vi "AP_2_pulse_control.vi"() -> ()   [LabVIEW 2023]
uses:
  <instrlib>/Quantum Composers 9000 Series/Public/Configure/Configure Chan Mode (Normal).vi
  <instrlib>/Quantum Composers 9000 Series/Quantum Composers 9000 Series.lvlib
panel:
  in  "Gas Pulse Enabled?":bool=TRUE
  in  "Mass Gate Enabled?":bool=TRUE
  in  "Initialization Type":string(combo)="Load from variables "
  in  "Load Conditions":bool
  in  "Save Conditions":bool
  in  "Detachment Laser On?":bool=TRUE
  in  "Detachment Laser Delay / us":dbl=500.0
  in  "Laser In Use":string(combo)="QuantaRay 170-30"
  in  "stop":bool
  in  "Mass Gate Width / us":dbl=0.5 format="%#_3f"
  in  "Mass Gate Delay / us":dbl=85.0
  in  "Repeller Delay / us":dbl=80.0
  # "AP2 Delay Controls"
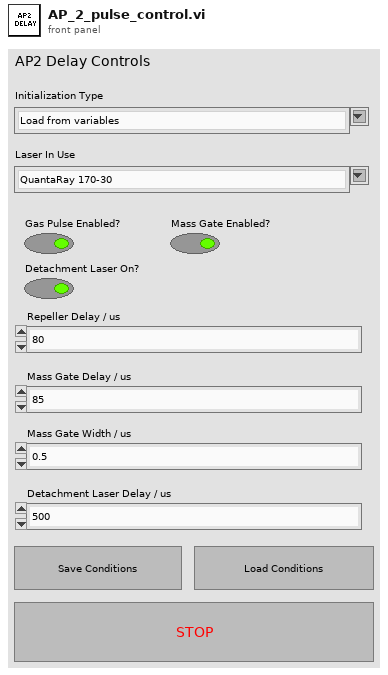
[diagram p1: front panel]
types:
  T1 = cluster{"Mass Gate Delay / us":refnum<vi>, "Mass Gate Width / us":refnum<vi>, "Repeller Delay / us":refnum<vi>, "Mass Gate Enabled?":refnum<vi>, "Gas Pulse Enabled?":refnum<vi>, "Detachment Laser On?":refnum<vi>, "Detachment Laser Delay / us":refnum<vi>}
  T2 = cluster{"Mass Gate Delay / us":dbl, "Mass Gate Width / us":dbl, "Repeller Delay / us":dbl, "Detachment Laser Delay / us":dbl, "Mass Gate Enabled?":bool, "Gas Pulse Enabled?":bool, "Detachment Laser On?":bool}
  T3 = enum16{"Disabled", "Pulse Inhibit", "Output Inhibit"}
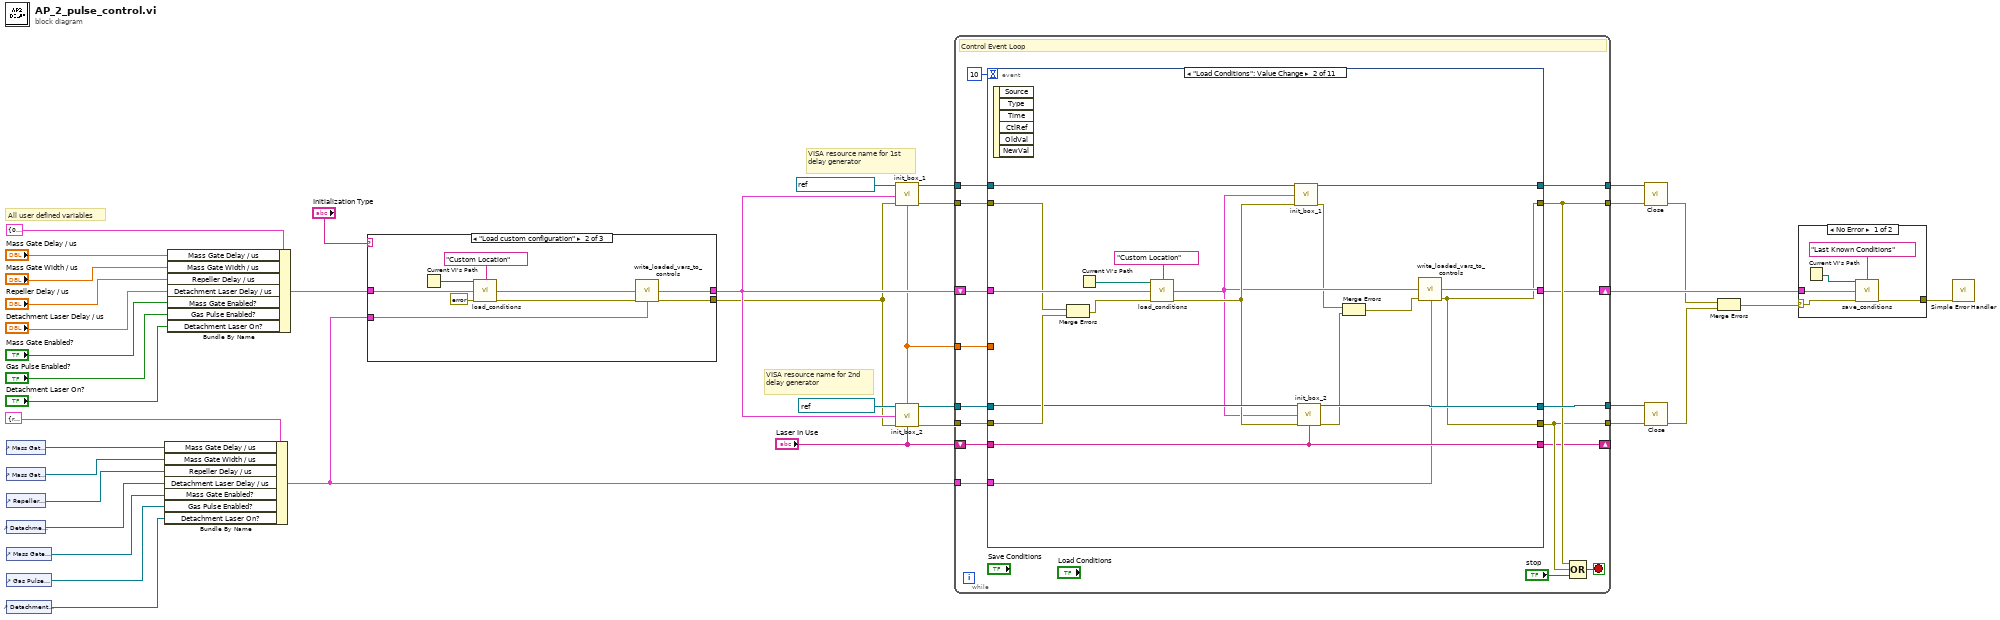
[diagram p0: block diagram]
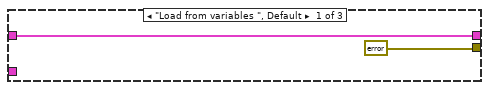
[diagram p2: hidden frame]
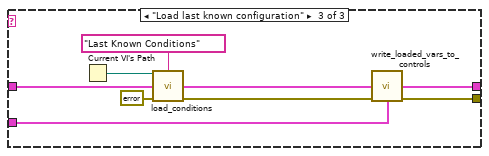
[diagram p3: hidden frame]
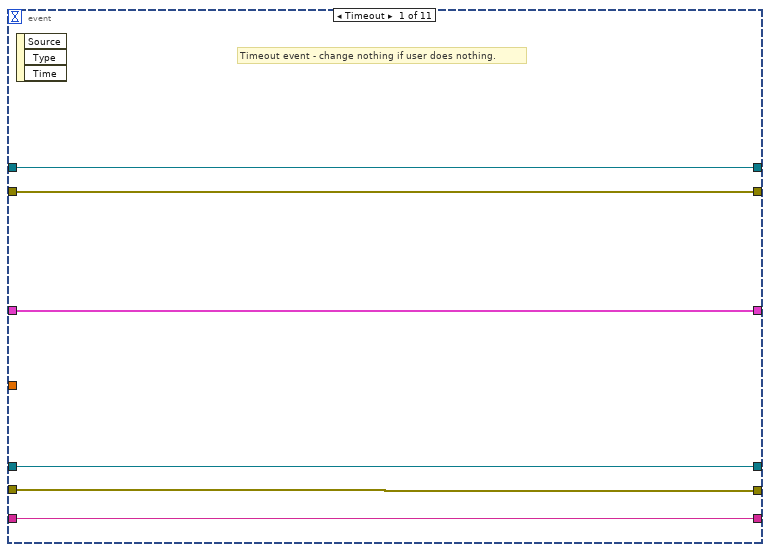
[diagram p5: hidden frame]
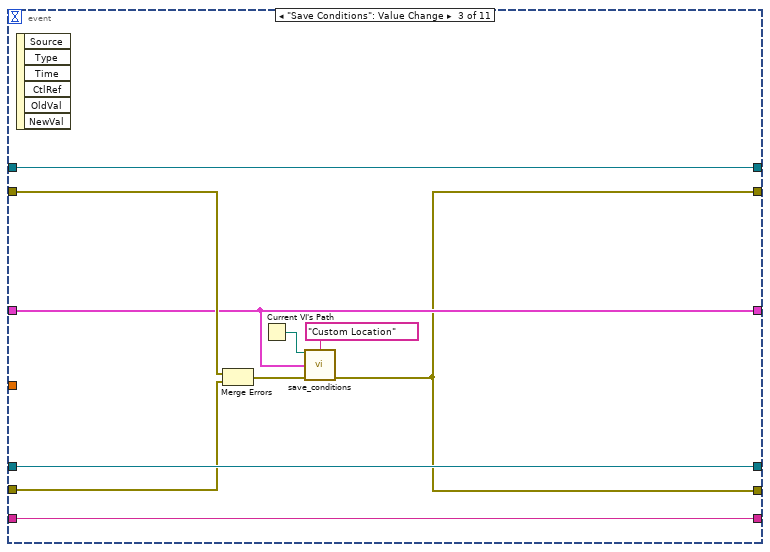
[diagram p6: hidden frame]
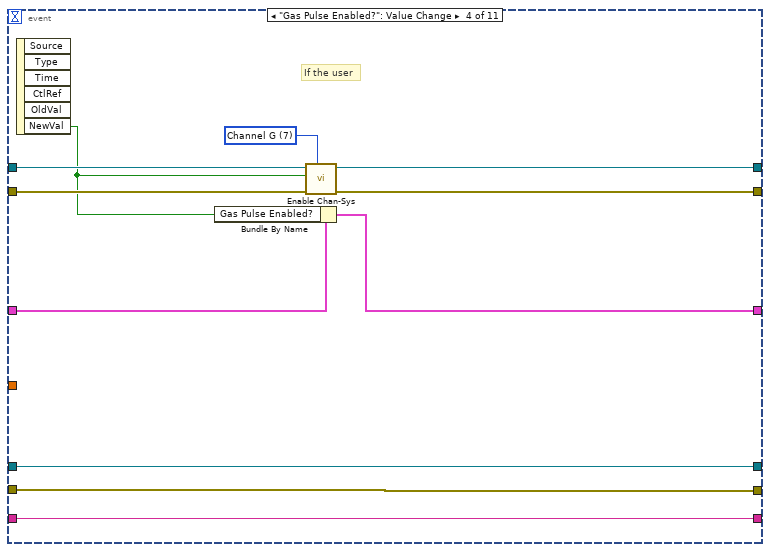
[diagram p7: hidden frame]
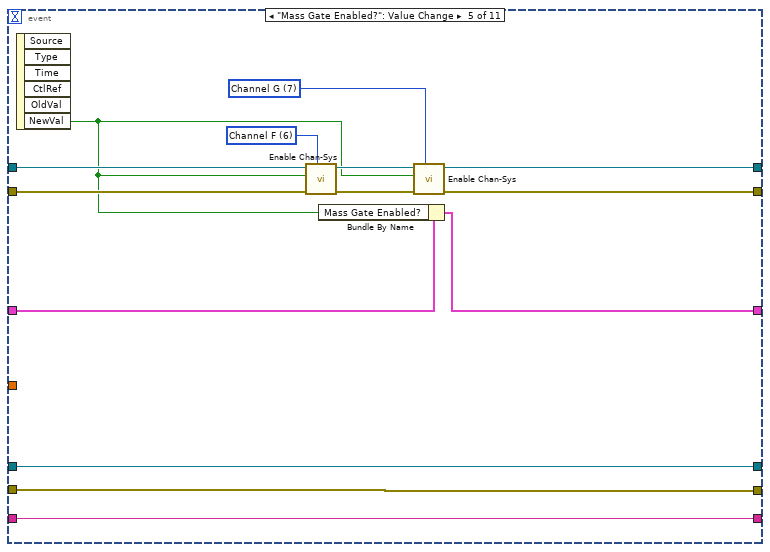
[diagram p8: hidden frame]
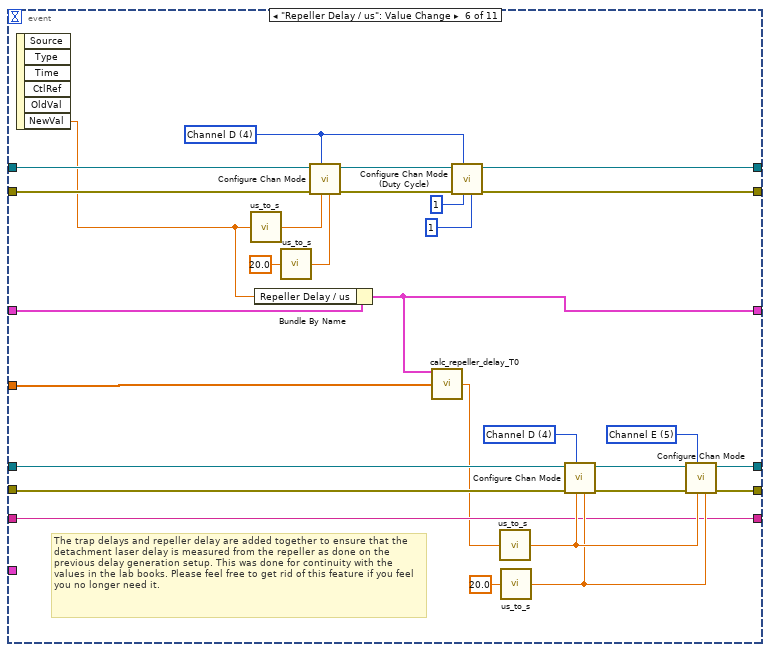
[diagram p9: hidden frame]
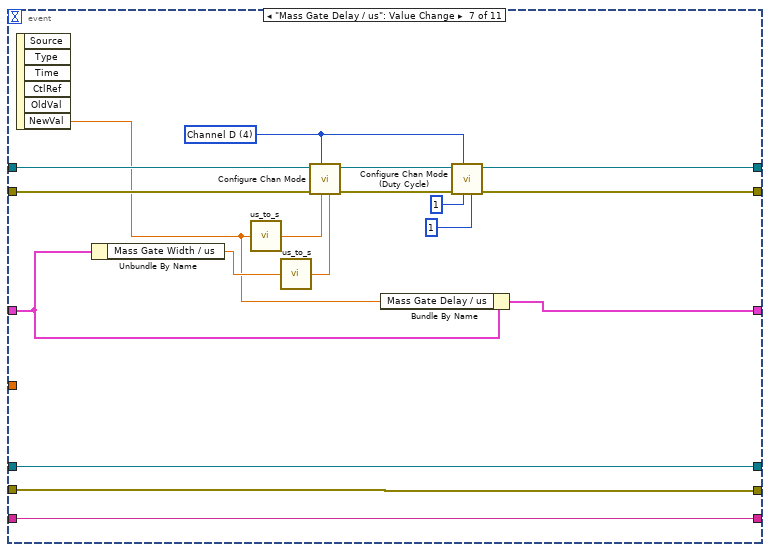
[diagram p10: hidden frame]
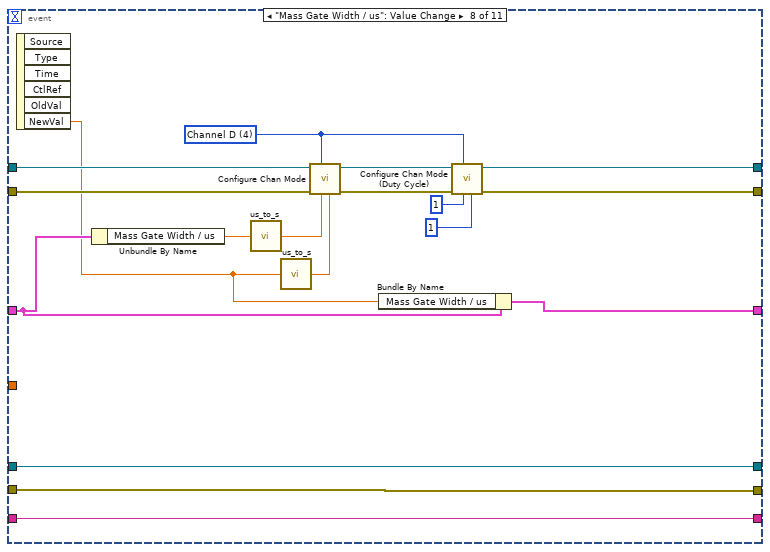
[diagram p11: hidden frame]
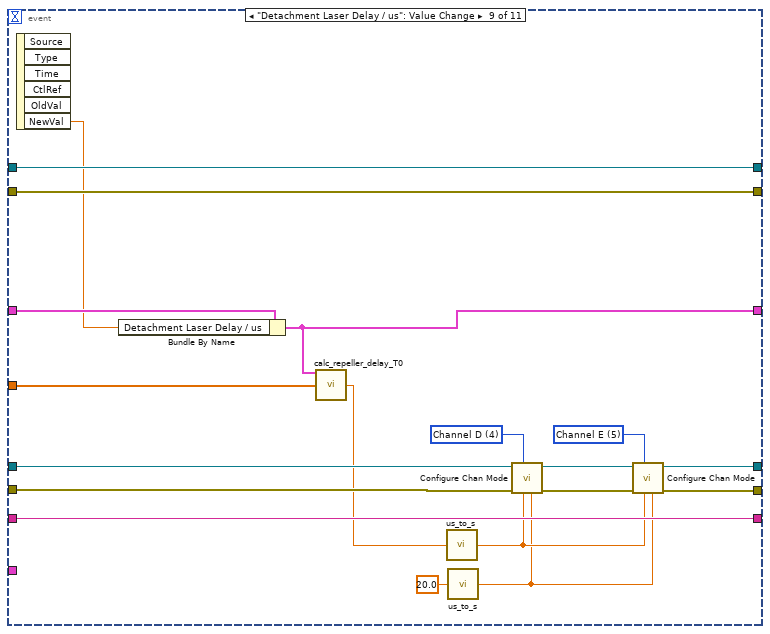
[diagram p12: hidden frame]
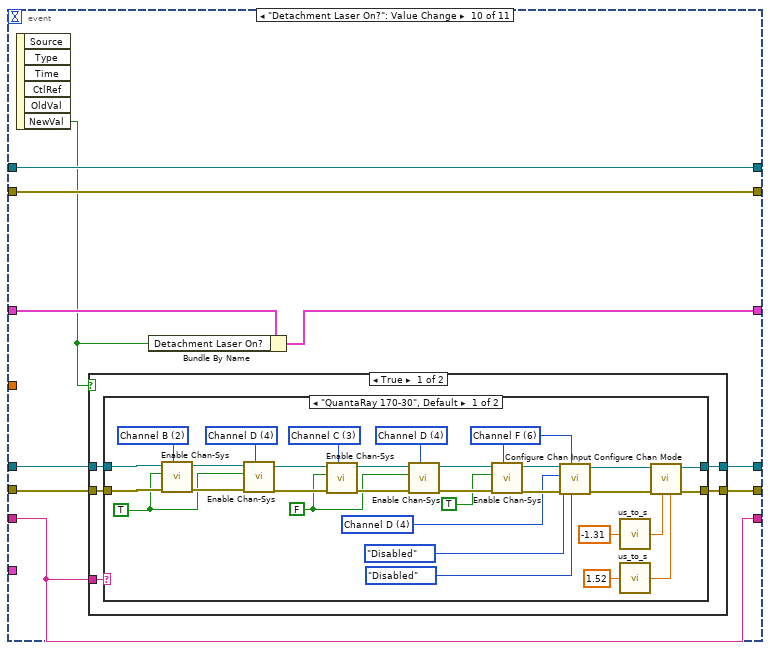
[diagram p13: hidden frame]
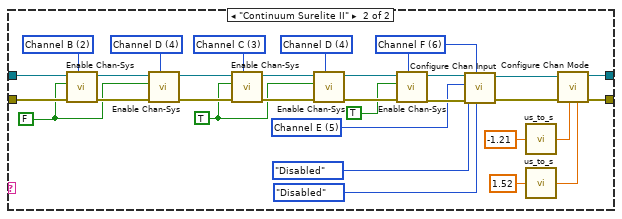
[diagram p14: hidden frame]
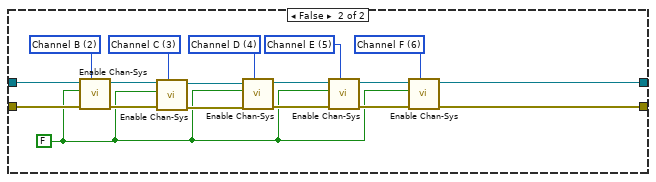
[diagram p15: hidden frame]
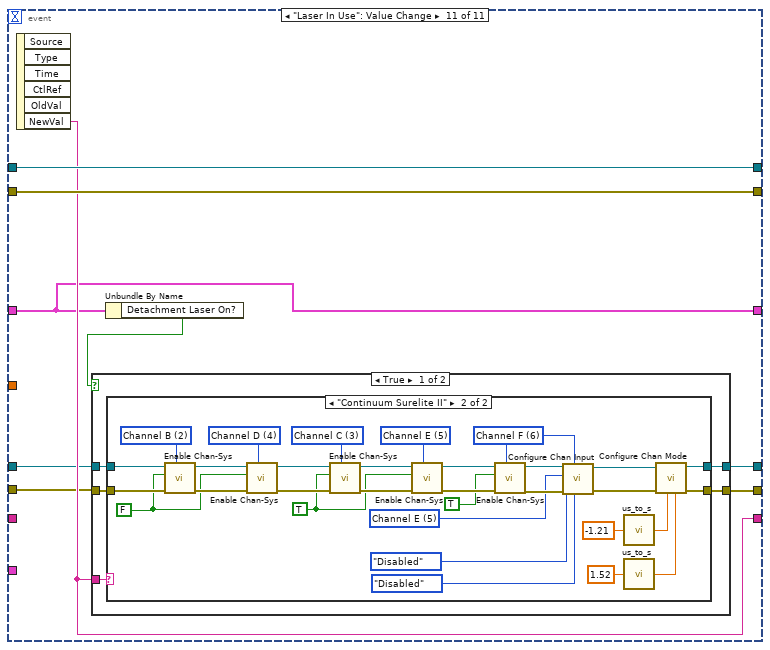
[diagram p16: hidden frame]
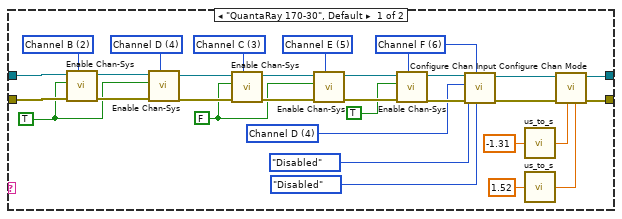
[diagram p17: hidden frame]
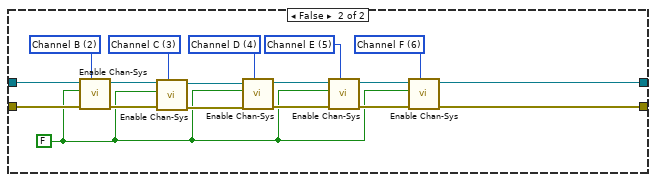
[diagram p18: hidden frame]
diagram:
  # "VISA resource name for 2nd delay generator"
  # "VISA resource name for 1st delay generator"
  # "All user defined variables"
  n1 = control-ref of="Mass Gate Delay / us"() -> (w12:refnum<vi>)
  n2 = control-ref of="Mass Gate Width / us"() -> (w11:refnum<vi>)
  n3 = control-ref of="Repeller Delay / us"() -> (w10:refnum<vi>)
  n4 = control-ref of="Detachment Laser Delay / us"() -> (w9:refnum<vi>)
  n5 = control-ref of="Mass Gate Enabled?"() -> (w2:refnum<vi>)
  n6 = control-ref of="Gas Pulse Enabled?"() -> (w1:refnum<vi>)
  n7 = control-ref of="Detachment Laser On?"() -> (w8:refnum<vi>)
  n8 = Bundle By Name(cluster=T1 {"Mass Gate Delay / us"=refnum, "Mass Gate Width / us"=refnum, "Repeller Delay / us"=refnum, "Mass Gate Enabled?"=refnum, "Gas Pulse Enabled?"=refnum, "Detachment Laser On?"=refnum, "Detachment Laser Delay / us"=refnum}, "Mass Gate Delay / us"=w12, "Mass Gate Width / us"=w11, "Repeller Delay / us"=w10, "Detachment Laser Delay / us"=w9, "Mass Gate Enabled?"=w2, "Gas Pulse Enabled?"=w1, "Detachment Laser On?"=w8) -> (w6:T1)
  n9 = Bundle By Name(cluster=T2 {"Mass Gate Delay / us"=0.0, "Mass Gate Width / us"=0.0, "Repeller Delay / us"=0.0, "Detachment Laser Delay / us"=500.0, "Mass Gate Enabled?"=TRUE, "Gas Pulse Enabled?"=TRUE, "Detachment Laser On?"=FALSE}, "Mass Gate Delay / us"="Mass Gate Delay / us", "Mass Gate Width / us"="Mass Gate Width / us", "Repeller Delay / us"="Repeller Delay / us", "Detachment Laser Delay / us"="Detachment Laser Delay / us", "Mass Gate Enabled?"="Mass Gate Enabled?", "Gas Pulse Enabled?"="Gas Pulse Enabled?", "Detachment Laser On?"="Detachment Laser On?") -> (w16:T2)
  n10 = case shown="\"Load custom configuration\"" "Initialization Type" {
    tunnel: w16 -> [w40 w49 w58]
    tunnel: [w40 w45 w54] -> w15
    tunnel: w6 -> [_ w46 w55]
    tunnel: [errorcluster {"status"=FALSE, "code"=0, "source"=""} ("error in") w43 w52] -> w7
    frame "Load from variables ", Default {
    }
    frame "Load custom configuration" {
      n11 = Current VI's Path() -> (path=w42:path)
      n12 = call "load_conditions.vi"("VI's Path"=w42, "Load Type"="Custom Location", "Config In"=w49, "error in"=errorcluster {"status"=FALSE, "code"=0, "source"=""}) -> ("Config Out"=w48:T2, "error out"=w47:errorcluster)  [unwired: 10 in]
      n13 = call "write_loaded_vars_to_controls.vi"("Variable Values"=w48, "error in (no error)"=w47, "Variable References"=w46) -> ("Variable Values Out"=w45:T2, "error out"=w43:errorcluster)  [unwired: 11 in]
    }
    frame "Load last known configuration" {
      n14 = Current VI's Path() -> (path=w51:path)
      n15 = call "load_conditions.vi"("VI's Path"=w51, "Load Type"="Last Known Conditions", "Config In"=w58, "error in"=errorcluster {"status"=FALSE, "code"=0, "source"=""}) -> ("Config Out"=w57:T2, "error out"=w56:errorcluster)  [unwired: 10 in]
      n16 = call "write_loaded_vars_to_controls.vi"("Variable Values"=w57, "error in (no error)"=w56, "Variable References"=w55) -> ("Variable Values Out"=w54:T2, "error out"=w52:errorcluster)  [unwired: 11 in]
    }
  }
  n17 = call "init_box_1.vi"("Box I VISA Name"=refnum<visa-resource-name> "QC_9530_DG1", "Controls Cluster"=w15, "error in (no error)"=w7) -> ("Box I VISA Name"=w34:refnum<visa-resource-name>, "Trap Delay Array"=w5:dbl[], "error out"=w33:errorcluster)  [unwired: 10 in]
  n18 = call "init_box_2.vi"("Box 2 VISA Name"=refnum<visa-resource-name> "QC_9530_DG2" ("Box I VISA Name"), "Trap Delay Array"=w5, "Controls Cluster"=w15, "error in (no error)"=w7, "Laser In Use"="Laser In Use") -> ("Box 2 VISA Name Out"=w25:refnum<visa-resource-name>, "Error out"=w24:errorcluster)  [unwired: 9 in]
  n19 = while {
    tunnel: w34 -> [w75]
    tunnel: w33 -> [w74]
    tunnel: [w73] -> w38
    tunnel: [w68] -> w37
    tunnel: w25 -> [w71]
    tunnel: w24 -> [w70]
    tunnel: [w69] -> w36
    tunnel: [w67] -> w35
    shift-right: [w63] -> w21
    shift-left: w15 -> [w64]
    shift-right: [w61] -> _
    shift-left: "Laser In Use" -> [w62]
    tunnel: w6 -> [w60]
    tunnel: w5 -> [w59]
    stop <- w66 stop-if-true
    # "Control Event Loop"
    n20 = event shown="[1] \"Load Conditions\": Value Change" {
      selector: _ -> [_ _ _ _ _ _ _ _ _ _ _]
      dyn-events: _ -> [_ _ _ _ _ _ _ _ _ _ _]
      timeout: 10 -> [_ _ _ _ _ _ _ _ _ _ _]
      tunnel: w75 -> [w81 w99 w110 w118 w132 w164 w180 w198 w219 w229 w323]
      tunnel: w74 -> [w80 w98 w106 w117 w131 w163 w179 w197 w218 w228 w322]
      tunnel: [w81 w91 w110 w116 w125 w160 w176 w194 w219 w229 w323] -> w73
      tunnel: [w80 w84 w101 w115 w124 w159 w175 w193 w218 w228 w322] -> w68
      tunnel: w71 -> [w79 w94 w109 w121 w135 w144 w182 w200 w217 w224 w318]
      tunnel: w70 -> [w78 w97 w107 w120 w134 w143 w181 w199 w216 w223 w317]
      tunnel: [w79 w95 w109 w121 w135 w142 w182 w200 w207 w222 w321] -> w69
      tunnel: [w78 w84 w101 w120 w134 w141 w181 w199 w206 w221 w320] -> w67
      tunnel: w64 -> [w77 w100 w104 w114 w130 w138 w169 w187 w214 w227 w315]
      tunnel: [w77 w90 w104 w113 w129 w136 w168 w186 w202 w226 w315] -> w63
      tunnel: w62 -> [w76 w92 w108 w119 w133 w140 w165 w183 w215 w220 _]
      tunnel: [w76 w92 w108 w119 w133 w140 w165 w183 w215 w220 w319] -> w61
      tunnel: w60 -> [_ w85 _ _ _ _ _ _ _ _ _]
      tunnel: w59 -> [_ _ _ _ _ w139 _ _ w203 _ _]
      event Timeout {
        # "Timeout event - change nothing if user does nothing."
        n21 = event-data() -> ()  [unwired: 1 in, 3 out]
      }
      event "Load Conditions": Value Change {
        n22 = event-data() -> ()  [unwired: 1 in, 6 out]
        n23 = Merge Errors(w98, w97) -> (w96:errorcluster)
        n24 = Current VI's Path() -> (path=w83:path)
        n25 = call "load_conditions.vi"("VI's Path"=w83, "Load Type"="Custom Location", "Config In"=w100, "error in"=w96) -> ("Config Out"=w89:T2, "error out"=w93:errorcluster)  [unwired: 10 in]
        n26 = call "init_box_1.vi"("Box I VISA Name"=w99, "Controls Cluster"=w89, "error in (no error)"=w93) -> ("Box I VISA Name"=w91:refnum<visa-resource-name>, "error out"=w88:errorcluster)  [unwired: 10 in, 1 out]
        n27 = call "init_box_2.vi"("Box 2 VISA Name"=w94, "Controls Cluster"=w89, "error in (no error)"=w93, "Laser In Use"=w92) -> ("Box 2 VISA Name Out"=w95:refnum<visa-resource-name>, "Error out"=w87:errorcluster)  [unwired: 10 in]
        n28 = Merge Errors(w88, w87) -> (w86:errorcluster)
        n29 = call "write_loaded_vars_to_controls.vi"("Variable Values"=w89, "error in (no error)"=w86, "Variable References"=w85) -> ("Variable Values Out"=w90:T2, "error out"=w84:errorcluster)  [unwired: 11 in]
      }
      event "Save Conditions": Value Change {
        n30 = event-data() -> ()  [unwired: 1 in, 6 out]
        n31 = Merge Errors(w106, w107) -> (w105:errorcluster)
        n32 = Current VI's Path() -> (path=w103:path)
        n33 = call "save_conditions.vi"("VI's Path"=w103, "Load Type"="Custom Location" ("Combo Box"), "output cluster"=w104, "error in"=w105) -> ("error out"=w101:errorcluster)  [unwired: 11 in]
      }
      event "Gas Pulse Enabled?": Value Change {
        w111 = 7 items=["System (To)", "Channel A", "Channel B", "Channel C", "Channel D", "Channel E", "Channel F", "Channel G", "Channel H"] ("Channel (1:Chan A)")
        # "If the user"
        n34 = event-data() -> ("NewVal"=w112:bool)  [unwired: 1 in, 5 out]
        n35 = Bundle By Name(cluster=w114, "Gas Pulse Enabled?"=w112) -> (w113:T2)
        n36 = call <instrlib>:"Enable Chan-Sys.vi"("Channel (1:Chan A)"=w111, "error in (no error)"=w117, "State (T:Enabled)"=w112, "VISA resource name"=w118) -> ("error out"=w115:errorcluster, "VISA resource name out"=w116:refnum<visa-resource-name>)  [unwired: 6 in]
      }
      event "Mass Gate Enabled?": Value Change {
        w122 = 7 items=["System (To)", "Channel A", "Channel B", "Channel C", "Channel D", "Channel E", "Channel F", "Channel G", "Channel H"] ("Channel (1:Chan A)")
        w128 = 6 items=["System (To)", "Channel A", "Channel B", "Channel C", "Channel D", "Channel E", "Channel F", "Channel G", "Channel H"] ("Channel (1:Chan A)")
        n37 = event-data() -> ("NewVal"=w123:bool)  [unwired: 1 in, 5 out]
        n38 = call <instrlib>:"Enable Chan-Sys.vi"("Channel (1:Chan A)"=w128, "error in (no error)"=w131, "State (T:Enabled)"=w123, "VISA resource name"=w132) -> ("error out"=w126:errorcluster, "VISA resource name out"=w127:refnum<visa-resource-name>)  [unwired: 6 in]
        n39 = Bundle By Name(cluster=w130, "Mass Gate Enabled?"=w123) -> (w129:T2)
        n40 = call <instrlib>:"Enable Chan-Sys.vi"("Channel (1:Chan A)"=w122, "error in (no error)"=w126, "State (T:Enabled)"=w123, "VISA resource name"=w127) -> ("error out"=w124:errorcluster, "VISA resource name out"=w125:refnum<visa-resource-name>)  [unwired: 6 in]
      }
      event "Repeller Delay / us": Value Change {
        w149 = 5 items=["Channel A"=1, "Channel B"=2, "Channel C"=3, "Channel D"=4, "Channel E"=5, "Channel F"=6, "Channel G"=7, "Channel H"=8] ("Channel (1:Chan A)")
        w150 = 4 items=["Channel A"=1, "Channel B"=2, "Channel C"=3, "Channel D"=4, "Channel E"=5, "Channel F"=6, "Channel G"=7, "Channel H"=8] ("Channel (1:Chan A)")
        w156 = 4 items=["Channel A"=1, "Channel B"=2, "Channel C"=3, "Channel D"=4, "Channel E"=5, "Channel F"=6, "Channel G"=7, "Channel H"=8] ("Channel (1:Chan A)")
        # "The trap delays and repeller delay are added together to ensure that the detachment laser delay is measured from the repeller as done on the previous delay generation setup. This was done for continuity with the values in the lab books. Please feel free to get rid of this feature if you feel you no longer need it."
        n41 = event-data() -> ("NewVal"=w152:dbl)  [unwired: 1 in, 5 out]
        n42 = call "us_to_s.vi"("Time / us"=w152) -> ("Time / s"=w155:dbl)
        n43 = Bundle By Name(cluster=w138, "Repeller Delay / us"=w152) -> (w136:T2)
        n44 = call "us_to_s.vi"("Time / us"=20.0) -> ("Time / s"=w153:dbl)
        n45 = call-poly <instrlib>:"Configure Chan Mode.vi"("Width (10 msec)"=w153, "Delay (10 msec)"=w155, "Channel (1:Chan A)"=w156, "error in (no error)"=w163, "VISA resource name"=w164) -> ("error out"=w161:errorcluster, "VISA resource name out"=w162:refnum<visa-resource-name>)  [unwired: 5 in]
        n46 = call "calc_repeller_delay_T0.vi"("Variable Values Out"=w136, "Trap Delay Array"=w139) -> ("Total Repeller Delay / us"=w137:dbl)  [unwired: 13 in]
        n47 = call <instrlib>:"Configure Chan Mode (Duty Cycle).vi"("Chan DC Off (10)"=1, "Chan DC On (10)"=1, "Channel (1:Chan A)"=w156, "error in (no error)"=w161, "VISA resource name"=w162) -> ("error out"=w159:errorcluster, "VISA resource name out"=w160:refnum<visa-resource-name>)  [unwired: 5 in]
        n48 = call "us_to_s.vi"("Time / us"=w137) -> ("Time / s"=w146:dbl)
        n49 = call "us_to_s.vi"("Time / us"=20.0) -> ("Time / s"=w145:dbl)
        n50 = call-poly <instrlib>:"Configure Chan Mode.vi"("Width (10 msec)"=w145, "Delay (10 msec)"=w146, "Channel (1:Chan A)"=w150, "error in (no error)"=w143, "VISA resource name"=w144) -> ("error out"=w147:errorcluster, "VISA resource name out"=w148:refnum<visa-resource-name>)  [unwired: 5 in]
        n51 = call-poly <instrlib>:"Configure Chan Mode.vi"("Width (10 msec)"=w145, "Delay (10 msec)"=w146, "Channel (1:Chan A)"=w149, "error in (no error)"=w147, "VISA resource name"=w148) -> ("error out"=w141:errorcluster, "VISA resource name out"=w142:refnum<visa-resource-name>)  [unwired: 5 in]
      }
      event "Mass Gate Delay / us": Value Change {
        w172 = 4 items=["Channel A"=1, "Channel B"=2, "Channel C"=3, "Channel D"=4, "Channel E"=5, "Channel F"=6, "Channel G"=7, "Channel H"=8] ("Channel (1:Chan A)")
        n52 = event-data() -> ("NewVal"=w166:dbl)  [unwired: 1 in, 5 out]
        n53 = Unbundle By Name(w169) -> ("Mass Gate Width / us"=w167:dbl)
        n54 = call "us_to_s.vi"("Time / us"=w166) -> ("Time / s"=w171:dbl)
        n55 = call "us_to_s.vi"("Time / us"=w167) -> ("Time / s"=w170:dbl)
        n56 = call-poly <instrlib>:"Configure Chan Mode.vi"("Width (10 msec)"=w170, "Delay (10 msec)"=w171, "Channel (1:Chan A)"=w172, "error in (no error)"=w179, "VISA resource name"=w180) -> ("error out"=w177:errorcluster, "VISA resource name out"=w178:refnum<visa-resource-name>)  [unwired: 5 in]
        n57 = Bundle By Name(cluster=w169, "Mass Gate Delay / us"=w166) -> (w168:T2)
        n58 = call <instrlib>:"Configure Chan Mode (Duty Cycle).vi"("Chan DC Off (10)"=1, "Chan DC On (10)"=1, "Channel (1:Chan A)"=w172, "error in (no error)"=w177, "VISA resource name"=w178) -> ("error out"=w175:errorcluster, "VISA resource name out"=w176:refnum<visa-resource-name>)  [unwired: 5 in]
      }
      event "Mass Gate Width / us": Value Change {
        w190 = 4 items=["Channel A"=1, "Channel B"=2, "Channel C"=3, "Channel D"=4, "Channel E"=5, "Channel F"=6, "Channel G"=7, "Channel H"=8] ("Channel (1:Chan A)")
        n59 = event-data() -> ("NewVal"=w184:dbl)  [unwired: 1 in, 5 out]
        n60 = Unbundle By Name(w187) -> ("Mass Gate Width / us"=w185:dbl)
        n61 = call "us_to_s.vi"("Time / us"=w185) -> ("Time / s"=w189:dbl)
        n62 = call "us_to_s.vi"("Time / us"=w184) -> ("Time / s"=w188:dbl)
        n63 = call-poly <instrlib>:"Configure Chan Mode.vi"("Width (10 msec)"=w188, "Delay (10 msec)"=w189, "Channel (1:Chan A)"=w190, "error in (no error)"=w197, "VISA resource name"=w198) -> ("error out"=w195:errorcluster, "VISA resource name out"=w196:refnum<visa-resource-name>)  [unwired: 5 in]
        n64 = Bundle By Name(cluster=w187, "Mass Gate Width / us"=w184) -> (w186:T2)
        n65 = call <instrlib>:"Configure Chan Mode (Duty Cycle).vi"("Chan DC Off (10)"=1, "Chan DC On (10)"=1, "Channel (1:Chan A)"=w190, "error in (no error)"=w195, "VISA resource name"=w196) -> ("error out"=w193:errorcluster, "VISA resource name out"=w194:refnum<visa-resource-name>)  [unwired: 5 in]
      }
      event "Detachment Laser Delay / us": Value Change {
        w210 = 5 items=["Channel A"=1, "Channel B"=2, "Channel C"=3, "Channel D"=4, "Channel E"=5, "Channel F"=6, "Channel G"=7, "Channel H"=8] ("Channel (1:Chan A)")
        w211 = 4 items=["Channel A"=1, "Channel B"=2, "Channel C"=3, "Channel D"=4, "Channel E"=5, "Channel F"=6, "Channel G"=7, "Channel H"=8] ("Channel (1:Chan A)")
        n66 = event-data() -> ("NewVal"=w213:dbl)  [unwired: 1 in, 5 out]
        n67 = Bundle By Name(cluster=w214, "Detachment Laser Delay / us"=w213) -> (w202:T2)
        n68 = call "calc_repeller_delay_T0.vi"("Variable Values Out"=w202, "Trap Delay Array"=w203) -> ("Total Repeller Delay / us"=w201:dbl)  [unwired: 13 in]
        n69 = call "us_to_s.vi"("Time / us"=w201) -> ("Time / s"=w205:dbl)
        n70 = call "us_to_s.vi"("Time / us"=20.0) -> ("Time / s"=w204:dbl)
        n71 = call-poly <instrlib>:"Configure Chan Mode.vi"("Width (10 msec)"=w204, "Delay (10 msec)"=w205, "Channel (1:Chan A)"=w211, "error in (no error)"=w216, "VISA resource name"=w217) -> ("error out"=w208:errorcluster, "VISA resource name out"=w209:refnum<visa-resource-name>)  [unwired: 5 in]
        n72 = call-poly <instrlib>:"Configure Chan Mode.vi"("Width (10 msec)"=w204, "Delay (10 msec)"=w205, "Channel (1:Chan A)"=w210, "error in (no error)"=w208, "VISA resource name"=w209) -> ("error out"=w206:errorcluster, "VISA resource name out"=w207:refnum<visa-resource-name>)  [unwired: 5 in]
      }
      event "Detachment Laser On?": Value Change {
        n73 = event-data() -> ("NewVal"=w225:bool)  [unwired: 1 in, 5 out]
        n74 = case shown="True" w225 {
          tunnel: w224 -> [w233 w314]
          tunnel: w223 -> [w232 w313]
          tunnel: [w231 w312] -> w222
          tunnel: [w230 w311] -> w221
          tunnel: w220 -> [w234 _]
          frame True {
            n75 = case shown="\"QuantaRay 170-30\", Default" w234 {
              tunnel: w233 -> [w265 w296]
              tunnel: w232 -> [w264 w295]
              tunnel: [w240 w271] -> w231
              tunnel: [w239 w270] -> w230
              frame "QuantaRay 170-30", Default {
                w244 = FALSE ("State (T:Enabled)")
                w245 = TRUE ("State (T:Enabled)")
                w246 = 4 items=["System (To)", "Channel A", "Channel B", "Channel C", "Channel D", "Channel E", "Channel F", "Channel G", "Channel H"] ("Channel (1:Chan A)")
                w247 = 2 items=["System (To)", "Channel A", "Channel B", "Channel C", "Channel D", "Channel E", "Channel F", "Channel G", "Channel H"] ("Channel (1:Chan A)")
                w248 = 3 items=["System (To)", "Channel A", "Channel B", "Channel C", "Channel D", "Channel E", "Channel F", "Channel G", "Channel H"] ("Channel (1:Chan A)")
                w251 = 4 items=["System (To)", "Channel A", "Channel B", "Channel C", "Channel D", "Channel E", "Channel F", "Channel G", "Channel H"] ("Sync Source (0:To)")
                w255 = 4 items=["System (To)", "Channel A", "Channel B", "Channel C", "Channel D", "Channel E", "Channel F", "Channel G", "Channel H"] ("Channel (1:Chan A)")
                w252 = 6 items=["System (To)", "Channel A", "Channel B", "Channel C", "Channel D", "Channel E", "Channel F", "Channel G", "Channel H"] ("Channel (1:Chan A)")
                n76 = call <instrlib>:"Enable Chan-Sys.vi"("Channel (1:Chan A)"=w247, "error in (no error)"=w264, "State (T:Enabled)"=w245, "VISA resource name"=w265) -> ("error out"=w262:errorcluster, "VISA resource name out"=w263:refnum<visa-resource-name>)  [unwired: 6 in]
                n77 = call <instrlib>:"Enable Chan-Sys.vi"("Channel (1:Chan A)"=w246, "error in (no error)"=w262, "State (T:Enabled)"=w245, "VISA resource name"=w263) -> ("error out"=w260:errorcluster, "VISA resource name out"=w261:refnum<visa-resource-name>)  [unwired: 6 in]
                n78 = call <instrlib>:"Enable Chan-Sys.vi"("Channel (1:Chan A)"=w248, "error in (no error)"=w260, "State (T:Enabled)"=w244, "VISA resource name"=w261) -> ("error out"=w258:errorcluster, "VISA resource name out"=w259:refnum<visa-resource-name>)  [unwired: 6 in]
                n79 = call <instrlib>:"Enable Chan-Sys.vi"("Channel (1:Chan A)"=w255, "error in (no error)"=w258, "State (T:Enabled)"=w244, "VISA resource name"=w259) -> ("error out"=w256:errorcluster, "VISA resource name out"=w257:refnum<visa-resource-name>)  [unwired: 6 in]
                n80 = call <instrlib>:"Enable Chan-Sys.vi"("Channel (1:Chan A)"=w252, "error in (no error)"=w256, "State (T:Enabled)"=TRUE, "VISA resource name"=w257) -> ("error out"=w253:errorcluster, "VISA resource name out"=w254:refnum<visa-resource-name>)  [unwired: 6 in]
                n81 = call <instrlib>:"Configure Chan Input.vi"("Gate Mode (0:Disabled)"=T3."Disabled", "Channel (1:Chan A)"=w252, "error in (no error)"=w253, "Gate Logic (0:Disabled)"=enum16{"Disabled", "Low", "High"}."Disabled", "Sync Source (0:To)"=w251, "VISA resource name"=w254) -> ("error out"=w241:errorcluster, "VISA resource name out"=w242:refnum<visa-resource-name>)  [unwired: 4 in]
                n82 = call "us_to_s.vi"("Time / us"=-1.31) -> ("Time / s"=w236:dbl)
                n83 = call "us_to_s.vi"("Time / us"=1.52) -> ("Time / s"=w235:dbl)
                n84 = call-poly <instrlib>:"Configure Chan Mode.vi"("Width (10 msec)"=w235, "Delay (10 msec)"=w236, "error in (no error)"=w241, "VISA resource name"=w242) -> ("error out"=w239:errorcluster, "VISA resource name out"=w240:refnum<visa-resource-name>)  [unwired: 6 in]
              }
              frame "Continuum Surelite II" {
                w275 = TRUE ("State (T:Enabled)")
                w276 = FALSE ("State (T:Enabled)")
                w277 = 4 items=["System (To)", "Channel A", "Channel B", "Channel C", "Channel D", "Channel E", "Channel F", "Channel G", "Channel H"] ("Channel (1:Chan A)")
                w278 = 2 items=["System (To)", "Channel A", "Channel B", "Channel C", "Channel D", "Channel E", "Channel F", "Channel G", "Channel H"] ("Channel (1:Chan A)")
                w279 = 3 items=["System (To)", "Channel A", "Channel B", "Channel C", "Channel D", "Channel E", "Channel F", "Channel G", "Channel H"] ("Channel (1:Chan A)")
                w282 = 5 items=["System (To)", "Channel A", "Channel B", "Channel C", "Channel D", "Channel E", "Channel F", "Channel G", "Channel H"] ("Sync Source (0:To)")
                w286 = 4 items=["System (To)", "Channel A", "Channel B", "Channel C", "Channel D", "Channel E", "Channel F", "Channel G", "Channel H"] ("Channel (1:Chan A)")
                w283 = 6 items=["System (To)", "Channel A", "Channel B", "Channel C", "Channel D", "Channel E", "Channel F", "Channel G", "Channel H"] ("Channel (1:Chan A)")
                n85 = call <instrlib>:"Enable Chan-Sys.vi"("Channel (1:Chan A)"=w278, "error in (no error)"=w295, "State (T:Enabled)"=w276, "VISA resource name"=w296) -> ("error out"=w293:errorcluster, "VISA resource name out"=w294:refnum<visa-resource-name>)  [unwired: 6 in]
                n86 = call <instrlib>:"Enable Chan-Sys.vi"("Channel (1:Chan A)"=w277, "error in (no error)"=w293, "State (T:Enabled)"=w276, "VISA resource name"=w294) -> ("error out"=w291:errorcluster, "VISA resource name out"=w292:refnum<visa-resource-name>)  [unwired: 6 in]
                n87 = call <instrlib>:"Enable Chan-Sys.vi"("Channel (1:Chan A)"=w279, "error in (no error)"=w291, "State (T:Enabled)"=w275, "VISA resource name"=w292) -> ("error out"=w289:errorcluster, "VISA resource name out"=w290:refnum<visa-resource-name>)  [unwired: 6 in]
                n88 = call <instrlib>:"Enable Chan-Sys.vi"("Channel (1:Chan A)"=w286, "error in (no error)"=w289, "State (T:Enabled)"=w275, "VISA resource name"=w290) -> ("error out"=w287:errorcluster, "VISA resource name out"=w288:refnum<visa-resource-name>)  [unwired: 6 in]
                n89 = call <instrlib>:"Enable Chan-Sys.vi"("Channel (1:Chan A)"=w283, "error in (no error)"=w287, "State (T:Enabled)"=TRUE, "VISA resource name"=w288) -> ("error out"=w284:errorcluster, "VISA resource name out"=w285:refnum<visa-resource-name>)  [unwired: 6 in]
                n90 = call <instrlib>:"Configure Chan Input.vi"("Gate Mode (0:Disabled)"=T3."Disabled", "Channel (1:Chan A)"=w283, "error in (no error)"=w284, "Gate Logic (0:Disabled)"=enum16{"Disabled", "Low", "High"}."Disabled", "Sync Source (0:To)"=w282, "VISA resource name"=w285) -> ("error out"=w272:errorcluster, "VISA resource name out"=w273:refnum<visa-resource-name>)  [unwired: 4 in]
                n91 = call "us_to_s.vi"("Time / us"=-1.21) -> ("Time / s"=w267:dbl)
                n92 = call "us_to_s.vi"("Time / us"=1.52) -> ("Time / s"=w266:dbl)
                n93 = call-poly <instrlib>:"Configure Chan Mode.vi"("Width (10 msec)"=w266, "Delay (10 msec)"=w267, "error in (no error)"=w272, "VISA resource name"=w273) -> ("error out"=w270:errorcluster, "VISA resource name out"=w271:refnum<visa-resource-name>)  [unwired: 6 in]
              }
            }
          }
          frame False {
            w298 = 6 items=["System (To)", "Channel A", "Channel B", "Channel C", "Channel D", "Channel E", "Channel F", "Channel G", "Channel H"] ("Channel (1:Chan A)")
            w299 = 5 items=["System (To)", "Channel A", "Channel B", "Channel C", "Channel D", "Channel E", "Channel F", "Channel G", "Channel H"] ("Channel (1:Chan A)")
            w300 = 4 items=["System (To)", "Channel A", "Channel B", "Channel C", "Channel D", "Channel E", "Channel F", "Channel G", "Channel H"] ("Channel (1:Chan A)")
            w301 = 3 items=["System (To)", "Channel A", "Channel B", "Channel C", "Channel D", "Channel E", "Channel F", "Channel G", "Channel H"] ("Channel (1:Chan A)")
            w297 = FALSE ("State (T:Enabled)")
            w302 = 2 items=["System (To)", "Channel A", "Channel B", "Channel C", "Channel D", "Channel E", "Channel F", "Channel G", "Channel H"] ("Channel (1:Chan A)")
            n94 = call <instrlib>:"Enable Chan-Sys.vi"("Channel (1:Chan A)"=w302, "error in (no error)"=w313, "State (T:Enabled)"=w297, "VISA resource name"=w314) -> ("error out"=w306:errorcluster, "VISA resource name out"=w310:refnum<visa-resource-name>)  [unwired: 6 in]
            n95 = call <instrlib>:"Enable Chan-Sys.vi"("Channel (1:Chan A)"=w301, "error in (no error)"=w306, "State (T:Enabled)"=w297, "VISA resource name"=w310) -> ("error out"=w305:errorcluster, "VISA resource name out"=w309:refnum<visa-resource-name>)  [unwired: 6 in]
            n96 = call <instrlib>:"Enable Chan-Sys.vi"("Channel (1:Chan A)"=w300, "error in (no error)"=w305, "State (T:Enabled)"=w297, "VISA resource name"=w309) -> ("error out"=w304:errorcluster, "VISA resource name out"=w308:refnum<visa-resource-name>)  [unwired: 6 in]
            n97 = call <instrlib>:"Enable Chan-Sys.vi"("Channel (1:Chan A)"=w299, "error in (no error)"=w304, "State (T:Enabled)"=w297, "VISA resource name"=w308) -> ("error out"=w303:errorcluster, "VISA resource name out"=w307:refnum<visa-resource-name>)  [unwired: 6 in]
            n98 = call <instrlib>:"Enable Chan-Sys.vi"("Channel (1:Chan A)"=w298, "error in (no error)"=w303, "State (T:Enabled)"=w297, "VISA resource name"=w307) -> ("error out"=w311:errorcluster, "VISA resource name out"=w312:refnum<visa-resource-name>)  [unwired: 6 in]
          }
        }
        n99 = Bundle By Name(cluster=w227, "Detachment Laser On?"=w225) -> (w226:T2)
      }
      event "Laser In Use": Value Change {
        n100 = event-data() -> ("NewVal"=w319:string)  [unwired: 1 in, 5 out]
        n101 = Unbundle By Name(w315) -> ("Detachment Laser On?"=w316:bool)
        n102 = case shown="True" w316 {
          tunnel: w318 -> [w327 w408]
          tunnel: w317 -> [w326 w407]
          tunnel: [w325 w406] -> w321
          tunnel: [w324 w405] -> w320
          tunnel: w319 -> [w328 _]
          frame True {
            n103 = case shown="\"Continuum Surelite II\"" w328 {
              tunnel: w327 -> [w359 w390]
              tunnel: w326 -> [w358 w389]
              tunnel: [w334 w365] -> w325
              tunnel: [w333 w364] -> w324
              frame "QuantaRay 170-30", Default {
                w338 = FALSE ("State (T:Enabled)")
                w339 = TRUE ("State (T:Enabled)")
                w340 = 4 items=["System (To)", "Channel A", "Channel B", "Channel C", "Channel D", "Channel E", "Channel F", "Channel G", "Channel H"] ("Channel (1:Chan A)")
                w341 = 2 items=["System (To)", "Channel A", "Channel B", "Channel C", "Channel D", "Channel E", "Channel F", "Channel G", "Channel H"] ("Channel (1:Chan A)")
                w342 = 3 items=["System (To)", "Channel A", "Channel B", "Channel C", "Channel D", "Channel E", "Channel F", "Channel G", "Channel H"] ("Channel (1:Chan A)")
                w345 = 4 items=["System (To)", "Channel A", "Channel B", "Channel C", "Channel D", "Channel E", "Channel F", "Channel G", "Channel H"] ("Sync Source (0:To)")
                w349 = 5 items=["System (To)", "Channel A", "Channel B", "Channel C", "Channel D", "Channel E", "Channel F", "Channel G", "Channel H"] ("Channel (1:Chan A)")
                w346 = 6 items=["System (To)", "Channel A", "Channel B", "Channel C", "Channel D", "Channel E", "Channel F", "Channel G", "Channel H"] ("Channel (1:Chan A)")
                n104 = call <instrlib>:"Enable Chan-Sys.vi"("Channel (1:Chan A)"=w341, "error in (no error)"=w358, "State (T:Enabled)"=w339, "VISA resource name"=w359) -> ("error out"=w356:errorcluster, "VISA resource name out"=w357:refnum<visa-resource-name>)  [unwired: 6 in]
                n105 = call <instrlib>:"Enable Chan-Sys.vi"("Channel (1:Chan A)"=w340, "error in (no error)"=w356, "State (T:Enabled)"=w339, "VISA resource name"=w357) -> ("error out"=w354:errorcluster, "VISA resource name out"=w355:refnum<visa-resource-name>)  [unwired: 6 in]
                n106 = call <instrlib>:"Enable Chan-Sys.vi"("Channel (1:Chan A)"=w342, "error in (no error)"=w354, "State (T:Enabled)"=w338, "VISA resource name"=w355) -> ("error out"=w352:errorcluster, "VISA resource name out"=w353:refnum<visa-resource-name>)  [unwired: 6 in]
                n107 = call <instrlib>:"Enable Chan-Sys.vi"("Channel (1:Chan A)"=w349, "error in (no error)"=w352, "State (T:Enabled)"=w338, "VISA resource name"=w353) -> ("error out"=w350:errorcluster, "VISA resource name out"=w351:refnum<visa-resource-name>)  [unwired: 6 in]
                n108 = call <instrlib>:"Enable Chan-Sys.vi"("Channel (1:Chan A)"=w346, "error in (no error)"=w350, "State (T:Enabled)"=TRUE, "VISA resource name"=w351) -> ("error out"=w347:errorcluster, "VISA resource name out"=w348:refnum<visa-resource-name>)  [unwired: 6 in]
                n109 = call <instrlib>:"Configure Chan Input.vi"("Gate Mode (0:Disabled)"=T3."Disabled", "Channel (1:Chan A)"=w346, "error in (no error)"=w347, "Gate Logic (0:Disabled)"=enum16{"Disabled", "Low", "High"}."Disabled", "Sync Source (0:To)"=w345, "VISA resource name"=w348) -> ("error out"=w335:errorcluster, "VISA resource name out"=w336:refnum<visa-resource-name>)  [unwired: 4 in]
                n110 = call "us_to_s.vi"("Time / us"=-1.31) -> ("Time / s"=w330:dbl)
                n111 = call "us_to_s.vi"("Time / us"=1.52) -> ("Time / s"=w329:dbl)
                n112 = call-poly <instrlib>:"Configure Chan Mode.vi"("Width (10 msec)"=w329, "Delay (10 msec)"=w330, "error in (no error)"=w335, "VISA resource name"=w336) -> ("error out"=w333:errorcluster, "VISA resource name out"=w334:refnum<visa-resource-name>)  [unwired: 6 in]
              }
              frame "Continuum Surelite II" {
                w369 = TRUE ("State (T:Enabled)")
                w370 = FALSE ("State (T:Enabled)")
                w371 = 4 items=["System (To)", "Channel A", "Channel B", "Channel C", "Channel D", "Channel E", "Channel F", "Channel G", "Channel H"] ("Channel (1:Chan A)")
                w372 = 2 items=["System (To)", "Channel A", "Channel B", "Channel C", "Channel D", "Channel E", "Channel F", "Channel G", "Channel H"] ("Channel (1:Chan A)")
                w373 = 3 items=["System (To)", "Channel A", "Channel B", "Channel C", "Channel D", "Channel E", "Channel F", "Channel G", "Channel H"] ("Channel (1:Chan A)")
                w376 = 5 items=["System (To)", "Channel A", "Channel B", "Channel C", "Channel D", "Channel E", "Channel F", "Channel G", "Channel H"] ("Sync Source (0:To)")
                w380 = 5 items=["System (To)", "Channel A", "Channel B", "Channel C", "Channel D", "Channel E", "Channel F", "Channel G", "Channel H"] ("Channel (1:Chan A)")
                w377 = 6 items=["System (To)", "Channel A", "Channel B", "Channel C", "Channel D", "Channel E", "Channel F", "Channel G", "Channel H"] ("Channel (1:Chan A)")
                n113 = call <instrlib>:"Enable Chan-Sys.vi"("Channel (1:Chan A)"=w372, "error in (no error)"=w389, "State (T:Enabled)"=w370, "VISA resource name"=w390) -> ("error out"=w387:errorcluster, "VISA resource name out"=w388:refnum<visa-resource-name>)  [unwired: 6 in]
                n114 = call <instrlib>:"Enable Chan-Sys.vi"("Channel (1:Chan A)"=w371, "error in (no error)"=w387, "State (T:Enabled)"=w370, "VISA resource name"=w388) -> ("error out"=w385:errorcluster, "VISA resource name out"=w386:refnum<visa-resource-name>)  [unwired: 6 in]
                n115 = call <instrlib>:"Enable Chan-Sys.vi"("Channel (1:Chan A)"=w373, "error in (no error)"=w385, "State (T:Enabled)"=w369, "VISA resource name"=w386) -> ("error out"=w383:errorcluster, "VISA resource name out"=w384:refnum<visa-resource-name>)  [unwired: 6 in]
                n116 = call <instrlib>:"Enable Chan-Sys.vi"("Channel (1:Chan A)"=w380, "error in (no error)"=w383, "State (T:Enabled)"=w369, "VISA resource name"=w384) -> ("error out"=w381:errorcluster, "VISA resource name out"=w382:refnum<visa-resource-name>)  [unwired: 6 in]
                n117 = call <instrlib>:"Enable Chan-Sys.vi"("Channel (1:Chan A)"=w377, "error in (no error)"=w381, "State (T:Enabled)"=TRUE, "VISA resource name"=w382) -> ("error out"=w378:errorcluster, "VISA resource name out"=w379:refnum<visa-resource-name>)  [unwired: 6 in]
                n118 = call <instrlib>:"Configure Chan Input.vi"("Gate Mode (0:Disabled)"=T3."Disabled", "Channel (1:Chan A)"=w377, "error in (no error)"=w378, "Gate Logic (0:Disabled)"=enum16{"Disabled", "Low", "High"}."Disabled", "Sync Source (0:To)"=w376, "VISA resource name"=w379) -> ("error out"=w366:errorcluster, "VISA resource name out"=w367:refnum<visa-resource-name>)  [unwired: 4 in]
                n119 = call "us_to_s.vi"("Time / us"=-1.21) -> ("Time / s"=w361:dbl)
                n120 = call "us_to_s.vi"("Time / us"=1.52) -> ("Time / s"=w360:dbl)
                n121 = call-poly <instrlib>:"Configure Chan Mode.vi"("Width (10 msec)"=w360, "Delay (10 msec)"=w361, "error in (no error)"=w366, "VISA resource name"=w367) -> ("error out"=w364:errorcluster, "VISA resource name out"=w365:refnum<visa-resource-name>)  [unwired: 6 in]
              }
            }
          }
          frame False {
            w392 = 6 items=["System (To)", "Channel A", "Channel B", "Channel C", "Channel D", "Channel E", "Channel F", "Channel G", "Channel H"] ("Channel (1:Chan A)")
            w393 = 5 items=["System (To)", "Channel A", "Channel B", "Channel C", "Channel D", "Channel E", "Channel F", "Channel G", "Channel H"] ("Channel (1:Chan A)")
            w394 = 4 items=["System (To)", "Channel A", "Channel B", "Channel C", "Channel D", "Channel E", "Channel F", "Channel G", "Channel H"] ("Channel (1:Chan A)")
            w395 = 3 items=["System (To)", "Channel A", "Channel B", "Channel C", "Channel D", "Channel E", "Channel F", "Channel G", "Channel H"] ("Channel (1:Chan A)")
            w391 = FALSE ("State (T:Enabled)")
            w396 = 2 items=["System (To)", "Channel A", "Channel B", "Channel C", "Channel D", "Channel E", "Channel F", "Channel G", "Channel H"] ("Channel (1:Chan A)")
            n122 = call <instrlib>:"Enable Chan-Sys.vi"("Channel (1:Chan A)"=w396, "error in (no error)"=w407, "State (T:Enabled)"=w391, "VISA resource name"=w408) -> ("error out"=w400:errorcluster, "VISA resource name out"=w404:refnum<visa-resource-name>)  [unwired: 6 in]
            n123 = call <instrlib>:"Enable Chan-Sys.vi"("Channel (1:Chan A)"=w395, "error in (no error)"=w400, "State (T:Enabled)"=w391, "VISA resource name"=w404) -> ("error out"=w399:errorcluster, "VISA resource name out"=w403:refnum<visa-resource-name>)  [unwired: 6 in]
            n124 = call <instrlib>:"Enable Chan-Sys.vi"("Channel (1:Chan A)"=w394, "error in (no error)"=w399, "State (T:Enabled)"=w391, "VISA resource name"=w403) -> ("error out"=w398:errorcluster, "VISA resource name out"=w402:refnum<visa-resource-name>)  [unwired: 6 in]
            n125 = call <instrlib>:"Enable Chan-Sys.vi"("Channel (1:Chan A)"=w393, "error in (no error)"=w398, "State (T:Enabled)"=w391, "VISA resource name"=w402) -> ("error out"=w397:errorcluster, "VISA resource name out"=w401:refnum<visa-resource-name>)  [unwired: 6 in]
            n126 = call <instrlib>:"Enable Chan-Sys.vi"("Channel (1:Chan A)"=w392, "error in (no error)"=w397, "State (T:Enabled)"=w391, "VISA resource name"=w401) -> ("error out"=w405:errorcluster, "VISA resource name out"=w406:refnum<visa-resource-name>)  [unwired: 6 in]
          }
        }
      }
    }
    n127 = Compound Arithmetic op=OR(w68, w67, "stop") -> (w66:bool)
  }
  n128 = call <instrlib>:"Close.vi"("error in (no error)"=w37, "VISA resource name"=w38) -> ("error out"=w19:errorcluster)  [unwired: 9 in]
  n129 = call <instrlib>:"Close.vi"("error in (no error)"=w35, "VISA resource name"=w36) -> ("error out"=w20:errorcluster)  [unwired: 9 in]
  n130 = Merge Errors(w19, w20) -> (w17:errorcluster)
  n131 = case shown="No Error" w17 {
    selector: w17 -> [w409 w414]
    tunnel: w21 -> [w413 _]
    tunnel: [w410 w414] -> w18
    frame No Error {
      n132 = Current VI's Path() -> (path=w412:path)
      n133 = call "save_conditions.vi"("VI's Path"=w412, "Load Type"="Last Known Conditions" ("Combo Box"), "output cluster"=w413, "error in"=w409) -> ("error out"=w410:errorcluster)  [unwired: 11 in]
    }
    frame Error {
    }
  }
  n134 = call <vilib>:"Simple Error Handler.vi"("error in (no error)"=w18) -> ()  [unwired: 4 in, 5 out]
